vi "Request DB obj.vi"(8 "error in (no error)":errorcluster, 11 "DB resource in":refnum<class "DB resource.lvclass">) -> (0 "error out":errorcluster, 3 "DB resource out":refnum<class "DB resource.lvclass">)   [LabVIEW 2020, in "DB resource interface.lvlib" / "DB resource.lvclass"]
uses:
  DB resource.lvclass
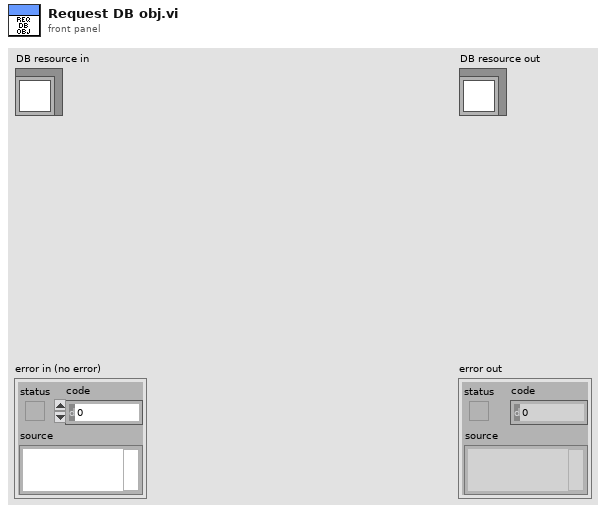
[diagram p1: front panel]
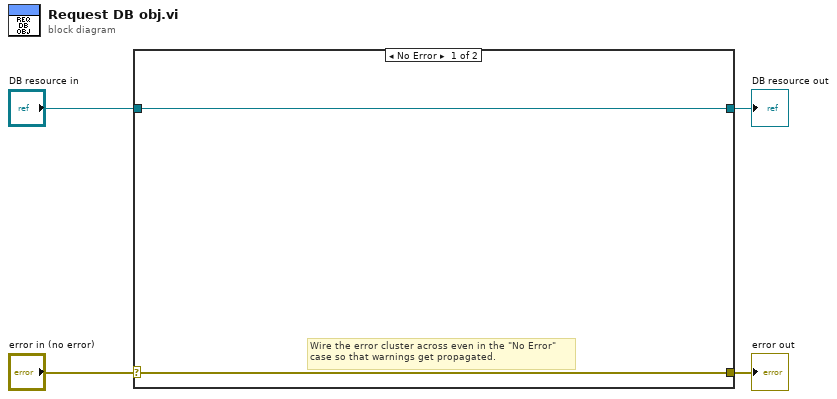
[diagram p0: block diagram]
diagram:
  n1 = case shown="No Error" "error in (no error)" {
    selector: "error in (no error)" -> [w5 w8]
    tunnel: [w5 w8] -> w3
    tunnel: [w6 w7] -> w1
    tunnel: "DB resource in" -> [w6 w7]
    frame No Error {
      # "Wire the error cluster across even in the \"No Error\"\ncase so that warnings get propagated."
    }
    frame Error {
    }
  }
  "error out" <- w3
  "DB resource out" <- w1
